vi "Send Error.vi"(8 "error in (no error)":errorcluster, 11 "Guardian in":refnum<class "Guardian.lvclass">) -> (0 "error out":errorcluster, 3 "Guardian out":refnum<class "Guardian.lvclass">)   [LabVIEW 2026, in "TALOS.lvlib" / "Guardian.lvlib" / "Guardian.lvclass"]
doc: "Use this VI to send an error to be processed by the Error Manager of the Distributed System.\n#What if the ASV update gives an error?"
uses:
  Guardian.lvclass
  Internal uServices/System uServices/Error Manager/Error Info.ctl
  Ancestor/Ancestor/Ancestor.lvclass/Ancestor.ctl
  Support VIs/Generate Error.vi
  FGV/Error Memory/Get Error Description.vi
  Ancestor/Ancestor/Read ID.vi
  Support VIs/Get Class Name.vi
  <vilib>/Utility/error.llb/Clear Errors.vi
  FGV/Error Memory/Error Memory Core.vi
  <vilib>/AdvancedString/Delimited String to 1D String Array.vi
  <vilib>/AdvancedString/Delimited String to 1D String Array (string).vi
  Support VIs/Circus Root Path.vi
  FGV/Error Memory/Error Crt Lvl checker.vi
  FGV/Error Memory/Error Memory Core.vi/40c8088d-b597-4017-91af-faa98e00292e.vi
  FGV/Error Memory/Error Memory Core.vi/d4a3ab98-063c-4e44-b43d-fbdcfe6c2be2.vi
  Support VIs/Global Memory.vi
  <vilib>/Utility/LVClass/Get LV Class Name.vi
  Support VIs/Is in Packed Library.vi
  Support VIs/TALOS Root path.vi
  Support VIs/Read CSV worksheet.vi
  Support VIs/Global Constants.vi
  <vilib>/Utility/error.llb/General Error Handler.vi
  Support VIs/Error Log.vi
  Ancestor/Ancestor/Ancestor.lvclass
  <vilib>/Comparison/Equal/Equal Functor/Equal Functor.lvclass
  Internal uServices/System uServices/Error Manager/Error Manager.lvclass
  TALOS.lvlib
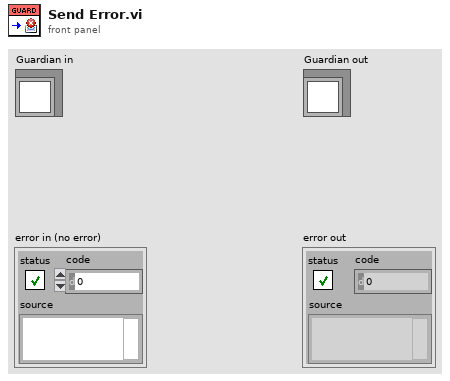
[diagram p1: front panel]
types:
  T1 = typedef "TALOS.lvlib/Error Manager.lvlib/Error Manager.lvclass/Error Info.ctl" = cluster{"error out":errorcluster, "Time Stamp":timestamp, "Machine Name":string, "GUID":string}
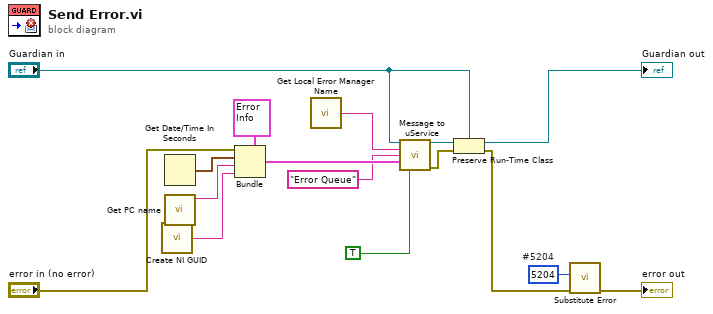
[diagram p0: block diagram]
diagram:
  w9 = 5204  # #5204
  n1 = call <vilib>:"Create NI GUID.vi"() -> ("NI GUID"=w12:string)
  n2 = Get Date/Time In Seconds() -> (seconds since 1Jan1904=w14:timestamp)
  n3 = call "Get PC name.vi"() -> ("Hostname"=w2:string)  [unwired: 10 in, 1 out]
  n4 = Bundle(cluster=T1 {"error out"={"status"=FALSE, "code"=0, "source"=""}, "Time Stamp"=timestamp(0 s since 1904-01-01), "Machine Name"="", "GUID"=""}, "error out"="error in (no error)", "Time Stamp"=w14, "Machine Name"=w2, "GUID"=w12) -> (w16:T1)
  n5 = call "Get Local Error Manager Name.vi"() -> ("Error Manager ID"=w1:string)  [unwired: 1 in]
  n6 = call "Message to uService.vi"("Guardian in"="Guardian in", "uService ID"=w1, "Message"="Error Queue", "Data"=w16, "Locale?"=TRUE) -> ("Guardian out"=w8:refnum<class "Guardian.lvclass">, "error out"=w4:errorcluster)  [unwired: 9 in]
  n7 = Preserve Run-Time Class(object in=w8, error in=w4, 2:"Guardian in") -> (object out=→"Guardian out":refnum<class "Guardian.lvclass">, error out=w5:errorcluster)
  n8 = call "Substitute Error.vi"("error in (no error)"=w5, "Error Code"=w9) -> ("error out"=→"error out":errorcluster)  [unwired: 9 in]
